vi "XNET Frame Property Node.vi"   [LabVIEW 2018]
doc: "Property node used to read/write properties for an XNET Frame I/O name."
uses:
  <resource>/objmgr/xnet.rc
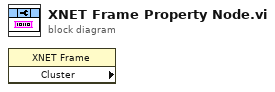
[diagram p0: block diagram]
diagram:
  n1 = property class="XNET Frame" props=["Cluster"]() -> ()  [unwired: 2 in, 3 out]
